vi "探头窗口-4-服务器版.vi"() -> ()   [LabVIEW 2013]
panel:
  in  "外部停止命令？":bool=TRUE
  out "引用-探头属性[]":refnum<vi>
  out "引用-监测模式？":refnum<vi>
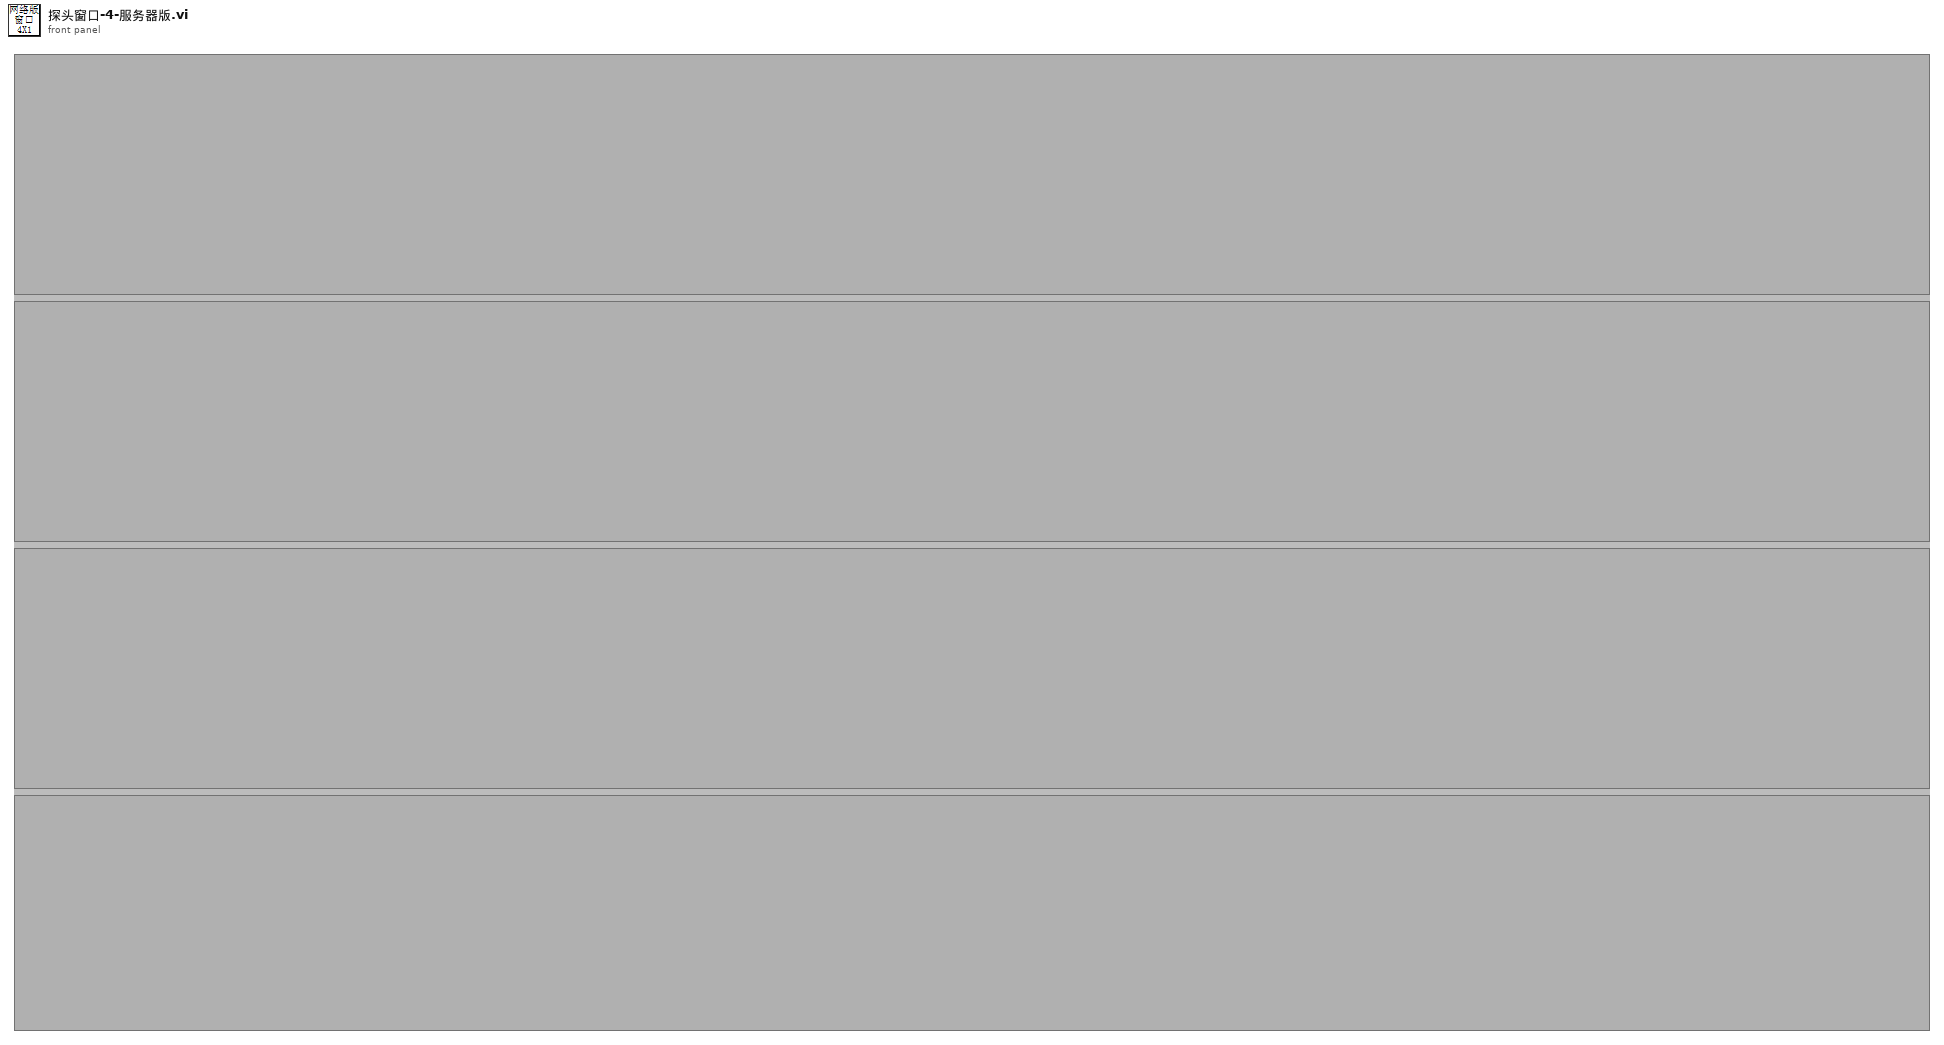
[diagram p1: front panel]
types:
  T1 = typedef "eventvkey.ctl" = enum16{"ASCII", "Enter", "Return", "Shift", "Ctrl", "Alt", "Cmd", "Opt", "Caps", "NumLock", "Clear", "Break", "Up", "Down", "Left", "Right", "Insert", "Delete", "Home", "End", "PageUp", "PageDown", "Escape", "Help", "Pause", "ScrollLock", "F1", "F2", "F3", "F4", "F5", "F6", "F7", "F8", "F9", "F10", "F11", "F12", "F13", "F14", "F15", "F16", "F17", "F18", "F19", "F20", "F21", "F22", "F23", "F24", "Play", "VolumeUp", "VolumeDown", "Mute", "Two Byte Char"}
  T2 = cluster{"探头地址与信息":cluster{"网络地址":cluster{"IP":string, "port":u16}, "探头信息":string}, "测量值":cluster{"时间":timestamp, "数值":dbl}, "限值":cluster{"限值1":dbl, "限值2":dbl}, "探头状态":enum16{"正常", "离线", "禁用", "一级报警", "二级报警"}}[]
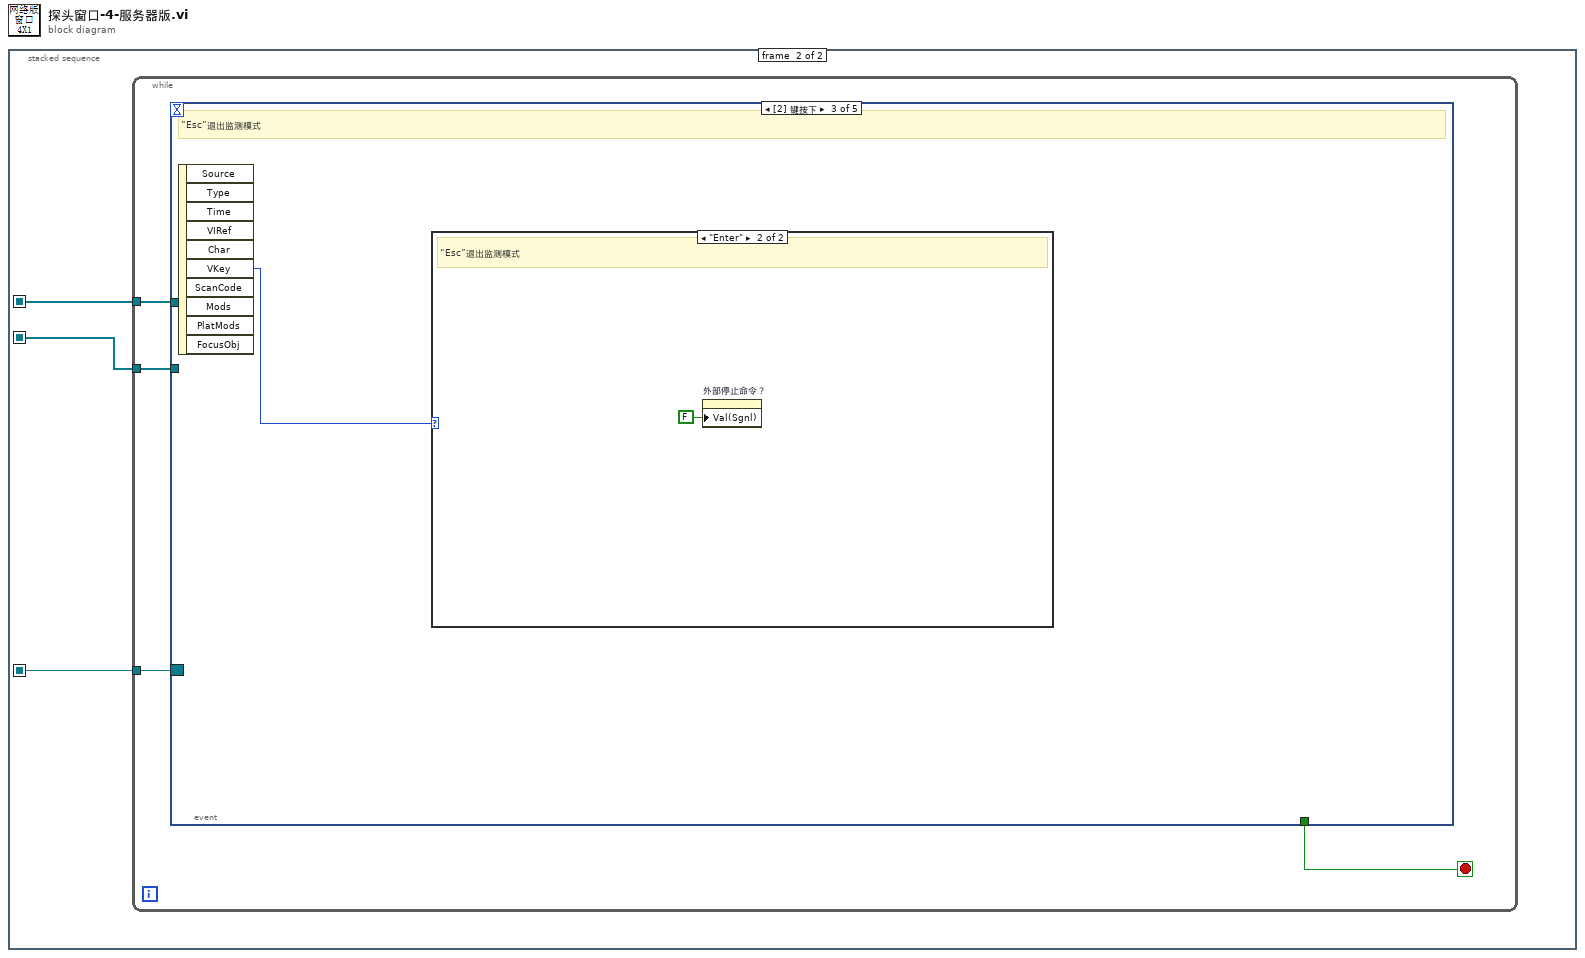
[diagram p0: block diagram]
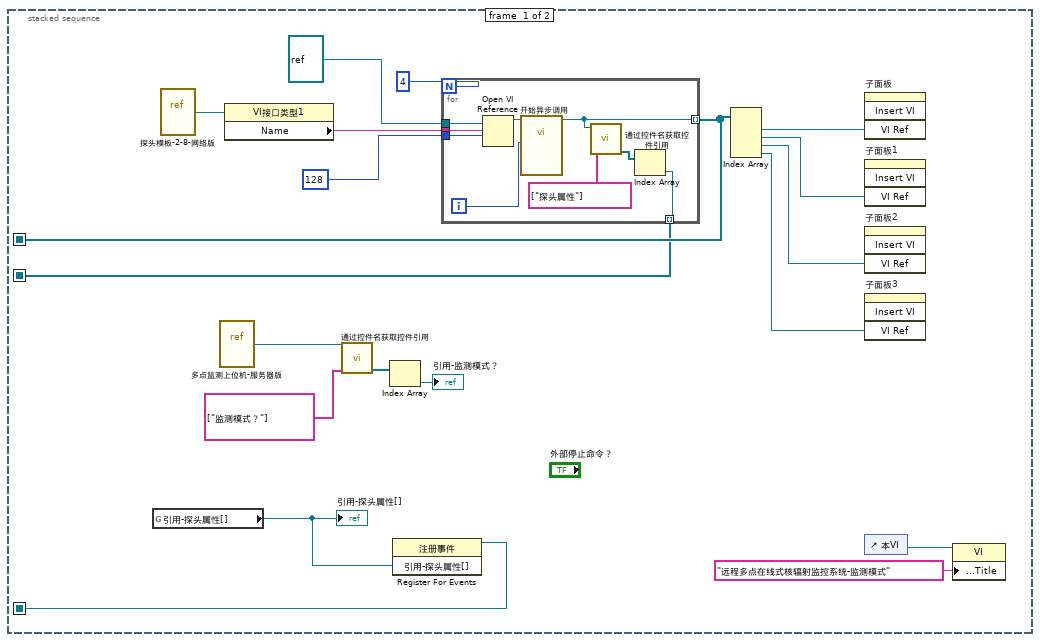
[diagram p2: hidden frame]
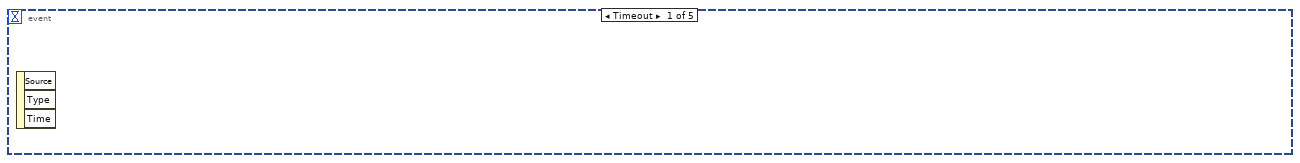
[diagram p3: hidden frame]
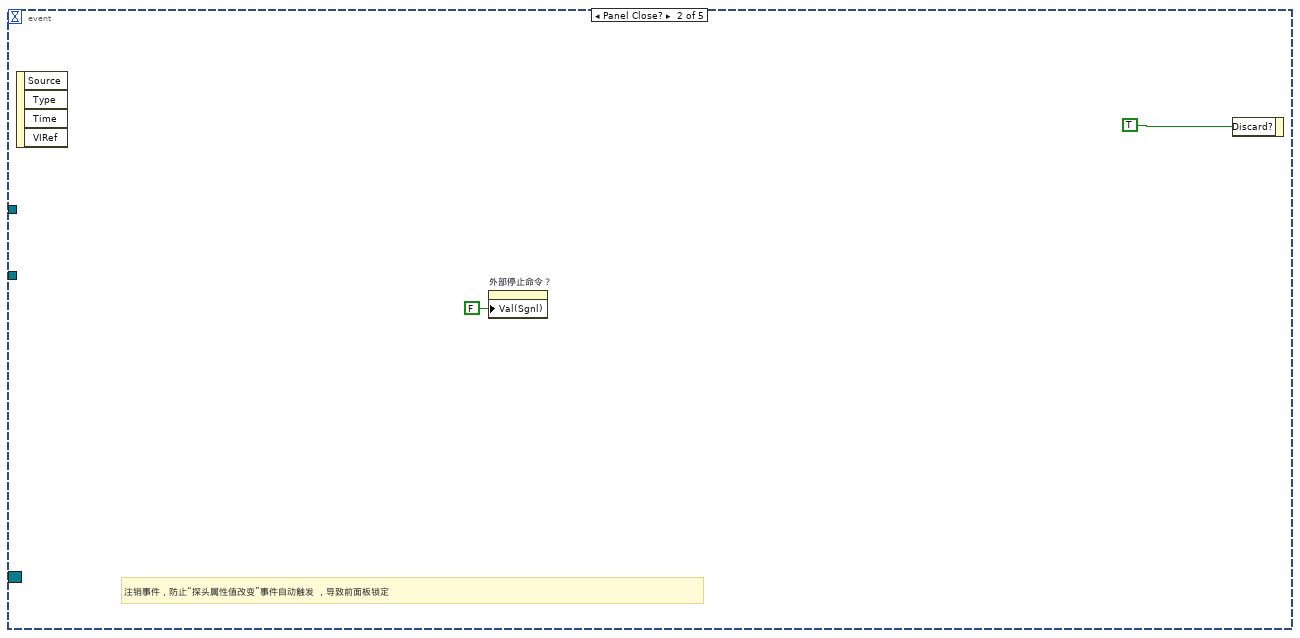
[diagram p4: hidden frame]
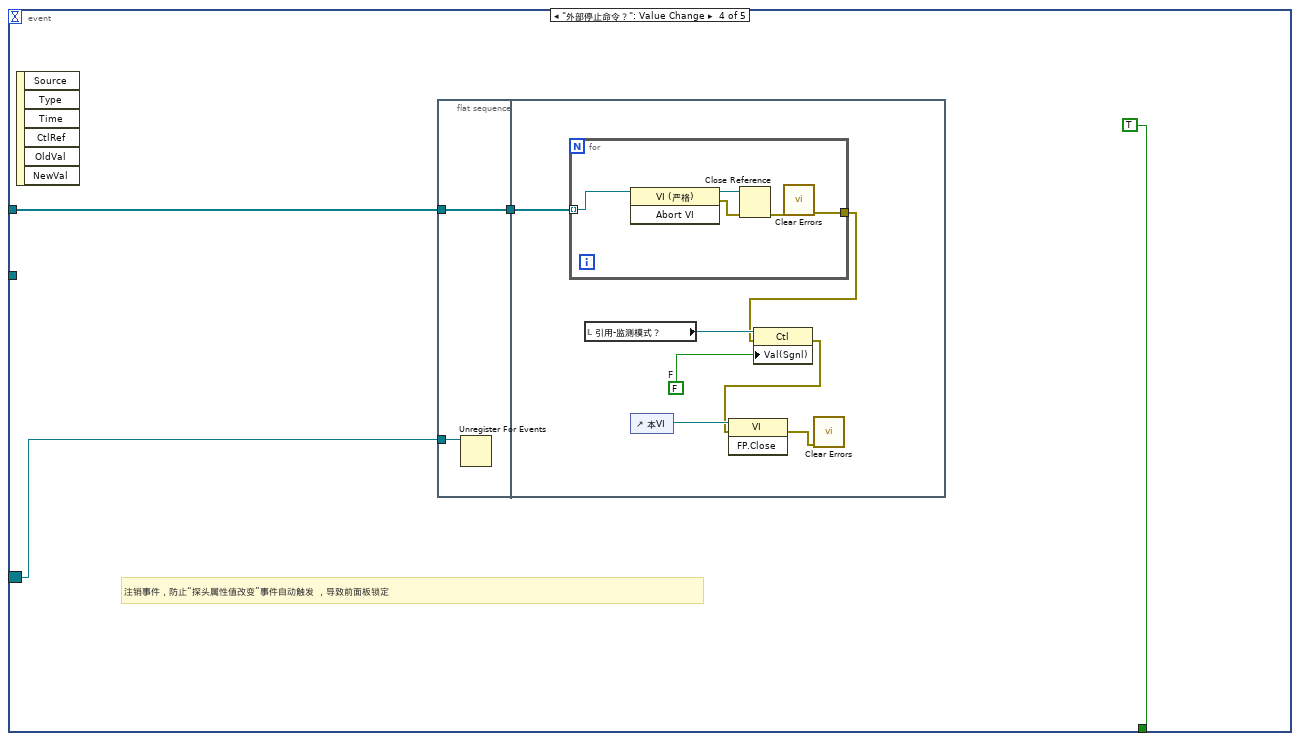
[diagram p6: hidden frame]
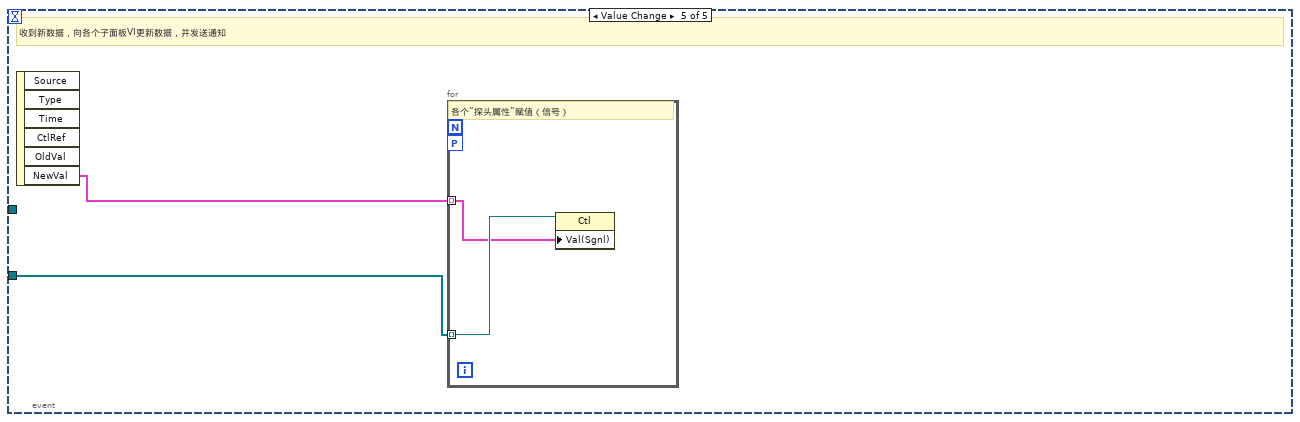
[diagram p7: hidden frame]
diagram:
  n1 = stacked-sequence {
    seq-local: [w15 _] -> [_ w31]
    seq-local: [w5 _] -> [_ w30]
    seq-local: [w3 _] -> [_ w29]
    frame #0 {
      n2 = global read "全局变量-35点监测.vi" "引用-探头属性[]"() -> (w4:refnum<vi>)
      "引用-探头属性[]" <- w4
      n3 = vi-ref "探头模板-2-8-网络版.vi"() -> (w19:refnum<vi>)
      n4 = vi-ref "多点监测上位机-服务器版.vi"() -> (w6:refnum<vi>)
      n5 = property class="VI接口类型1"(reference=w19) -> ("Name"=w18:string)  [unwired: 1 in, 2 out]
      n6 = call "通过控件名获取控件引用.vi"("控件名数组"=string[] ["监测模式？"], "VI引用"=w6) -> ("控件引用输出"=w8:refnum<vi>[])  [unwired: 7 in, 2 out]
      n7 = Index Array(array=w8) -> (element=→"引用-监测模式？":refnum<vi>)  [unwired: 1 in]
      n8 = register-events(w4) -> (reference out=w3:refnum<event-registration>)  [unwired: 2 in, 1 out]
      n9 = for {
        N: 4 -> [_]
        tunnel: w18 -> [w28]
        tunnel: 128 ("选项") -> [w27]
        tunnel: refnum<vi> refnum ("类型说明符VI引用句柄（仅用于类型）") -> [w26]
        tunnel: [w21] -> w15 mode=indexing
        tunnel: [w22] -> w5 mode=indexing
        i -> [w20]
        n10 = Open VI Reference(type specifier VI Refnum (for type only)=w26, vi path=w28, options=w27) -> (vi reference=w23:refnum<vi>)  [unwired: 3 in, 1 out]
        n11 = call-by-ref "开始异步调用"(reference=w23, "探头序号"=w20) -> (reference out=w21:refnum<vi>)  [unwired: 12 in, 1 out]
        n12 = call "通过控件名获取控件引用.vi"("控件名数组"=string[] ["探头属性"], "VI引用"=w21) -> ("控件引用输出"=w25:refnum<vi>[])  [unwired: 7 in, 2 out]
        n13 = Index Array(array=w25) -> (element=w22:refnum<vi>)  [unwired: 1 in]
      }
      n14 = Index Array(array=w15) -> (element #1=w14:refnum<vi>, element #2=w13:refnum<vi>, element #3=w12:refnum<vi>, element #4=w11:refnum<vi>)  [unwired: 4 in]
      n15 = invoke on="子面板" class="子面板" method="Insert VI"("VI Ref"=w14) -> ()  [unwired: 3 in, 4 out]
      n16 = invoke on="子面板1" class="SubPnl" method="Insert VI"("VI Ref"=w13) -> ()  [unwired: 3 in, 4 out]
      n17 = invoke on="子面板2" class="SubPnl" method="Insert VI"("VI Ref"=w12) -> ()  [unwired: 3 in, 4 out]
      n18 = invoke on="子面板3" class="SubPnl" method="Insert VI"("VI Ref"=w11) -> ()  [unwired: 3 in, 4 out]
      n19 = control-ref of="本VI"() -> (w2:refnum<vi>)
      n20 = property class="VI"(reference=w2, "Front Panel.Title"="远程多点在线式核辐射监控系统-监测模式" ("前面板窗口:标题")) -> ()  [unwired: 1 in, 2 out]
    }
    frame #1 {
      n21 = while {
        tunnel: w31 -> [w34]
        tunnel: w30 -> [w33]
        tunnel: w29 -> [w32]
        stop <- w35 stop-if-true
        n22 = event shown="[2] 键按下" {
          selector: w32 -> [_ _ _ w40 _]
          dyn-events: _ -> [_ _ _ _ _]
          timeout: _ -> [_ _ _ _ _]
          tunnel: [_ _ _ TRUE ("放弃？") _] -> w35
          tunnel: w34 -> [_ _ _ w42 _]
          tunnel: w33 -> [_ _ _ _ w58]
          event Timeout {
            n23 = event-data() -> ()  [unwired: 1 in, 3 out]
          }
          event Panel Close? {
            # "注销事件，防止“探头属性值改变”事件自动触发 ，导致前面板锁定"
            n24 = event-data() -> ()  [unwired: 1 in, 4 out]
            n25 = property on="外部停止命令？" class="Bool (严格)"("Val(Sgnl)"=FALSE ("值(信号)")) -> ()  [unwired: 2 in, 2 out]
            n26 = event-data("Discard?"=TRUE ("放弃？")) -> ()  [unwired: 1 in, 1 out]
          }
          event Key Down {
            # "“Esc”退出监测模式"
            n27 = event-data() -> ("VKey"=w38:T1)  [unwired: 1 in, 9 out]
            n28 = case shown="\"Enter\"" w38 {
              frame "ASCII", Default {
              }
              frame "Enter" {
                # "“Esc”退出监测模式"
                n29 = property on="外部停止命令？" class="Bool (严格)"("Val(Sgnl)"=FALSE ("值(信号)")) -> ()  [unwired: 2 in, 2 out]
              }
            }
          }
          event "外部停止命令？": Value Change {
            # "注销事件，防止“探头属性值改变”事件自动触发 ，导致前面板锁定"
            n30 = event-data() -> ()  [unwired: 1 in, 6 out]
            n31 = flat-sequence {
              tunnel: w42 -> [w45]
              tunnel: [w45] -> w41
              tunnel: w40 -> [w44]
              tunnel: w41 -> [w52]
              frame #0 {
                n32 = Unregister For Events(event registration refnum=w44) -> ()  [unwired: 1 in, 1 out]
              }
              frame #1 {
                w51 = FALSE  # F
                n33 = for {
                  tunnel: w52 -> [w57] mode=indexing
                  tunnel: [w53] -> w47
                  n34 = invoke class="VI (严格)" method="Abort VI"(reference=w57) -> (reference out=w55:refnum<vi>, error out=w56:errorcluster)  [unwired: 2 in, 1 out]
                  n35 = Close Reference(reference=w55, error in (no error)=w56) -> (error out=w54:errorcluster)
                  n36 = call <vilib>:"Clear Errors.vi"("error in (no error)"=w54) -> ("error out"=w53:errorcluster)  [unwired: 6 in]
                }
                n37 = local read "引用-监测模式？"() -> (w50:refnum<vi>)
                n38 = control-ref of="本VI"() -> (w49:refnum<vi>)
                n39 = property class="Ctl"(reference=w50, error in=w47, "Val(Sgnl)"=w51) -> (error out=w48:errorcluster)  [unwired: 1 out]
                n40 = invoke class="VI" method="FP.Close"(reference=w49, error in=w48) -> (error out=w46:errorcluster)  [unwired: 1 in, 2 out]
                n41 = call <vilib>:"Clear Errors.vi"("error in (no error)"=w46) -> ()  [unwired: 6 in, 1 out]
              }
            }
          }
          event Value Change {
            # "收到新数据，向各个子面板VI更新数据，并发送通知"
            n42 = event-data() -> ("NewVal"=w59:T2)  [unwired: 1 in, 5 out]
            n43 = for {
              workers-P: _ -> [_]
              tunnel: w58 -> [w61] mode=indexing
              tunnel: w59 -> [w60] mode=indexing
              # "各个“探头属性”赋值（信号）"
              n44 = property class="Ctl"(reference=w61, "Val(Sgnl)"=w60) -> ()  [unwired: 1 in, 2 out]
            }
          }
        }
      }
    }
  }
